vi "test Get Parameters.vi"(8 "error in":errorcluster, 11 "TestCase in":refnum<class "Scripting.lvclass">) -> (0 "error out":errorcluster, 3 "TestCase out":refnum<class "Scripting.lvclass">)   [LabVIEW 2020, in "Scripting.lvclass"]
uses:
  Scripting.lvclass
  C:/Program Files (x86)/National Instruments/LabVIEW 2020/vi.lib/addons/_JKI Toolkits/VI Tester/TestCase.llb/TestCase.lvclass
  <vilib>/addons/_JKI Toolkits/VI Tester/TestCase.llb/TestCase.lvclass
  Scripting/AIM/Constants.vi
  Scripting/AIM/AIM ARINC 429 Scripting.lvlib
  Scripting/ARINC 429/ARINC 429 Scripting.lvlib
  <vilib>/NI/NI VeriStand Encoding and Decoding/Encoding.ctl
  <vilib>/NI/NI VeriStand Encoding and Decoding/Encoding and Decoding.lvlib
  Shared/Parameter Definition.ctl
  <vilib>/NI VeriStand/Custom Device Tools/Custom Device Utility Library/Custom Device Utility Library.lvlib
  Shared/Label Properties.ctl
  <vilib>/NI VeriStand/Custom Device Tools/Custom Device Utility Library/NI VeriStand - Search for Item by GUID.vi
  <vilib>/NI VeriStand/Custom Device API/Custom Device API.lvlib
  Shared/Label.ctl
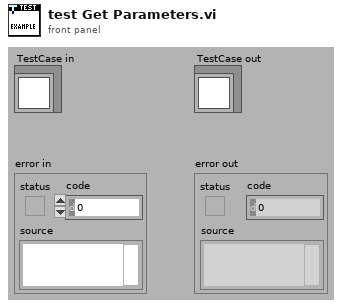
[diagram p1: front panel]
types:
  T1 = typedef "Label Properties.ctl" = cluster{"label (Dec)":T2, "SDI value":u8, "SDI enabled":bool}
  T2 = typedef "Label.ctl" = u8
  T3 = typedef "Parameter Definition.ctl" = cluster{"start index":i32, "size":i32, "encoding":T4, "signed":bool, "scale multiplier":dbl, "scale offset":dbl}
  T4 = typedef "Encoding and Decoding.lvlib/Encoding.ctl" = enum16{"BNR", "BCD", "Discrete"}
  T5 = typedef "Custom Device API.lvlib/Custom Device Item Ref.ctl" = u64
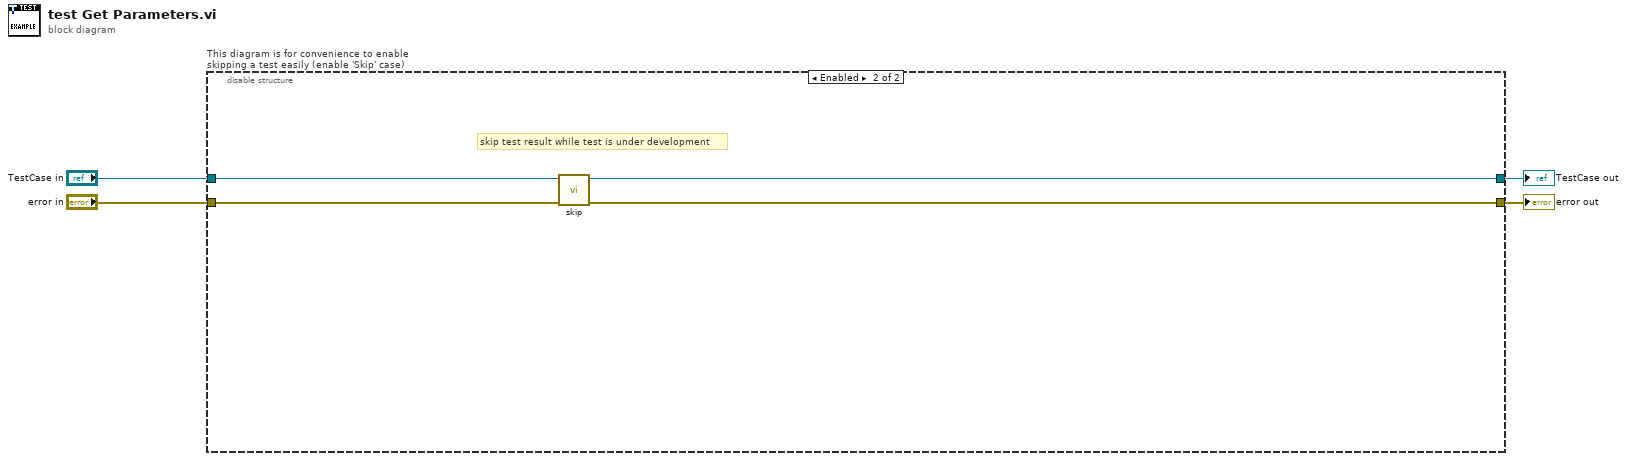
[diagram p0: block diagram]
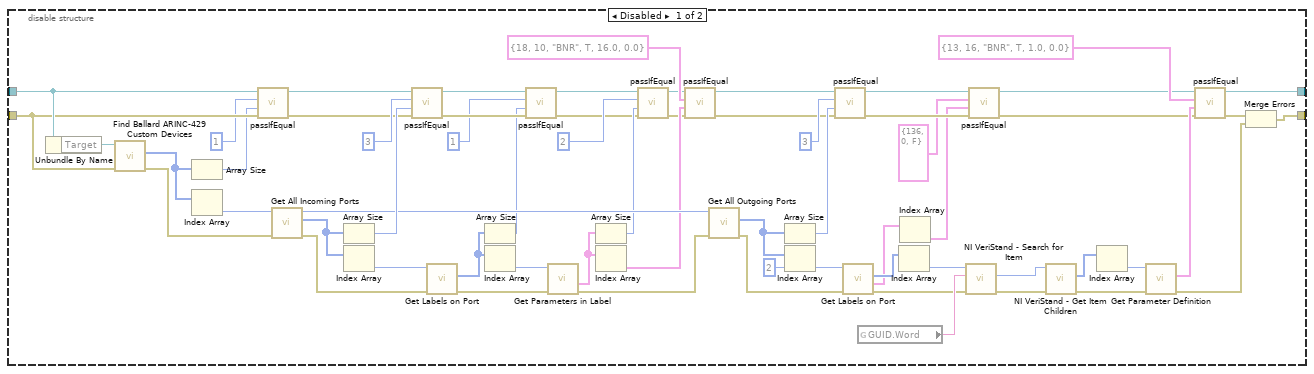
[diagram p2: hidden frame]
diagram:
  n1 = disable-structure "This diagram is for convenience to enable skipping a test easily (enable 'Skip' case)" shown="Enabled" {
    disable-tunnel: "TestCase in" -> [w64 w71]
    disable-tunnel: [w44 w69] -> w1
    disable-tunnel: [w46 w70] -> w3
    disable-tunnel: "error in" -> [w63 w68]
    frame Disabled {
      n2 = Unbundle By Name(w64) -> ("Target"=w66:refnum<k24>)
      n3 = call "Find Ballard ARINC-429 Custom Devices.vi"("error in"=w63, "target in"=w66) -> ("error out"=w55:errorcluster, "Ballard ARINC 429 custom devices"=w5:u64[])  [unwired: 7 in, 1 out]
      n4 = Array Size(array=w5) -> (size(s)=w61:i32)
      n5 = Index Array(array=w5) -> (element=w65:u64)  [unwired: 1 in]
      n6 = call-dynamic "passIfEqual.vi"("error in (no error)"=w63, "y"=w61, "x"=1 ("size(s)"), "TestCase in"=w64) -> ("error out"=w56:errorcluster, "TestCase out"=w57:refnum<class "Scripting.lvclass">)  [unwired: 6 in]
      n7 = call "Get All Incoming Ports.vi"("error in"=w55, "Ballard ARINC 429 custom device in"=w65) -> ("error out"=w25:errorcluster, "incoming ports"=w60:T5[], "Ballard ARINC 429 custom device out"=w54:T5)  [unwired: 7 in]
      n8 = Array Size(array=w60) -> (size(s)=w58:i32)
      n9 = Index Array(array=w60) -> (element=w27:T5)  [unwired: 1 in]
      n10 = call-dynamic "passIfEqual.vi"("error in (no error)"=w56, "y"=w58, "x"=3 ("size(s)"), "TestCase in"=w57) -> ("error out"=w38:errorcluster, "TestCase out"=w39:refnum<class "Scripting.lvclass">)  [unwired: 6 in]
      n11 = call "Get Labels on Port.vi"("error in"=w25, "port in"=w27) -> ("error out"=w24:errorcluster, "labels"=w26:T5[])  [unwired: 6 in, 2 out]
      n12 = Array Size(array=w26) -> (size(s)=w35:i32)
      n13 = Index Array(array=w26) -> (element=w37:T5)  [unwired: 1 in]
      n14 = call-dynamic "passIfEqual.vi"("error in (no error)"=w38, "y"=w35, "x"=1 ("size(s)"), "TestCase in"=w39) -> ("error out"=w30:errorcluster, "TestCase out"=w31:refnum<class "Scripting.lvclass">)  [unwired: 6 in]
      n15 = call "Get Parameters in Label.vi"("error in"=w24, "label in"=w37) -> ("error out"=w41:errorcluster, "parameter definitions"=w34:T3[])  [unwired: 6 in, 2 out]
      n16 = Array Size(array=w34) -> (size(s)=w32:i32)
      n17 = Index Array(array=w34) -> (element=w40:T3)  [unwired: 1 in]
      n18 = call-dynamic "passIfEqual.vi"("error in (no error)"=w30, "y"=w32, "x"=2 ("size(s)"), "TestCase in"=w31) -> ("error out"=w28:errorcluster, "TestCase out"=w29:refnum<class "Scripting.lvclass">)  [unwired: 6 in]
      n19 = call-dynamic "passIfEqual.vi"("error in (no error)"=w28, "y"=w40, "x"=T3 {"start index"=18, "size"=10, "encoding"=enum."BNR", "signed"=TRUE, "scale multiplier"=16.0, "scale offset"=0.0} ("parameter definition"), "TestCase in"=w29) -> ("error out"=w50:errorcluster, "TestCase out"=w51:refnum<class "Scripting.lvclass">)  [unwired: 6 in]
      n20 = call "Get All Outgoing Ports.vi"("error in"=w41, "Ballard ARINC 429 custom device in"=w54) -> ("error out"=w23:errorcluster, "outgoing ports"=w49:T5[])  [unwired: 7 in, 1 out]
      n21 = Array Size(array=w49) -> (size(s)=w52:i32)
      n22 = Index Array(array=w49, index=2) -> (element=w22:T5)
      n23 = call-dynamic "passIfEqual.vi"("error in (no error)"=w50, "y"=w52, "x"=3 ("size(s)"), "TestCase in"=w51) -> ("error out"=w16:errorcluster, "TestCase out"=w17:refnum<class "Scripting.lvclass">)  [unwired: 6 in]
      n24 = call "Get Labels on Port.vi"("error in"=w23, "port in"=w22) -> ("error out"=w18:errorcluster, "labels properties"=w13:T1[], "labels"=w21:T5[])  [unwired: 6 in, 1 out]
      n25 = global read "Constants.vi" "GUID.Word"() -> (w19:string)
      n26 = Index Array(array=w21) -> (element=w20:T5)  [unwired: 1 in]
      n27 = Index Array(array=w13) -> (element=w12:T1)  [unwired: 1 in]
      n28 = call-poly <vilib>:"NI VeriStand - Search for Item.vi"("error in"=w18, "Item GUID"=w19, "Section Ref in"=w20) -> ("error out"=w9:errorcluster, "Item Ref"=w10:T5)  [unwired: 5 in, 2 out]
      n29 = call-dynamic "passIfEqual.vi"("error in (no error)"=w16, "y"=w12, "x"=T1 {"label (Dec)"=136, "SDI value"=0, "SDI enabled"=FALSE} ("element"), "TestCase in"=w17) -> ("error out"=w14:errorcluster, "TestCase out"=w15:refnum<class "Scripting.lvclass">)  [unwired: 6 in]
      n30 = call <vilib>:"NI VeriStand - Get Item Children.vi"("error in (no error)"=w9, "Item Ref in"=w10) -> ("error out"=w8:errorcluster, "Child Refs"=w6:T5[])  [unwired: 6 in, 2 out]
      n31 = Index Array(array=w6) -> (element=w7:T5)  [unwired: 1 in]
      n32 = call "Get Parameter Definition.vi"("error in"=w8, "parameter ref in"=w7) -> ("error out"=w47:errorcluster, "parameter definition"=w45:T3)  [unwired: 7 in, 1 out]
      n33 = call-dynamic "passIfEqual.vi"("error in (no error)"=w14, "y"=w45, "x"=T3 {"start index"=13, "size"=16, "encoding"=enum."BNR", "signed"=TRUE, "scale multiplier"=1.0, "scale offset"=0.0} ("parameter definition"), "TestCase in"=w15) -> ("error out"=w43:errorcluster, "TestCase out"=w44:refnum<class "Scripting.lvclass">)  [unwired: 6 in]
      n34 = Merge Errors(w43, w47) -> (w46:errorcluster)
    }
    frame Enabled {
      # "skip test result while test is under development"
      n35 = call <vilib>:"skip.vi"("error in (no error)"=w68, "TestCase in"=w71) -> ("error out"=w70:errorcluster, "TestCase out"=w69:refnum<class "Scripting.lvclass">)  [unwired: 8 in]
    }
  }
  "error out" <- w3
  "TestCase out" <- w1
